vi "Conversion umToFs.vi"(8 "error in (no error)":errorcluster caption="entrée d'erreur (pas d'erreur)", 10 "um":dbl, 11 "UI SA en entrée":refnum<class "UI SmarAct.lvclass">) -> (0 "error out":errorcluster caption="sortie d'erreur", 2 "Fs":ext, 3 "UI SA en sortie":refnum<class "UI SmarAct.lvclass">)   [LabVIEW 2024, in "UI SmarAct.lvclass"]
uses:
  UI SmarAct.lvclass
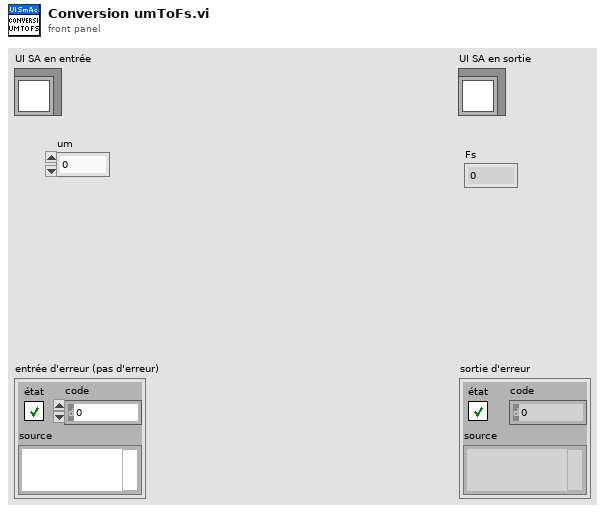
[diagram p1: front panel]
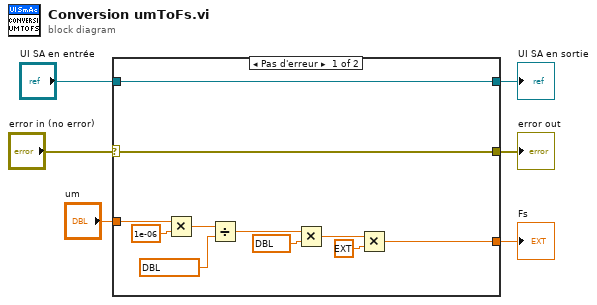
[diagram p0: block diagram]
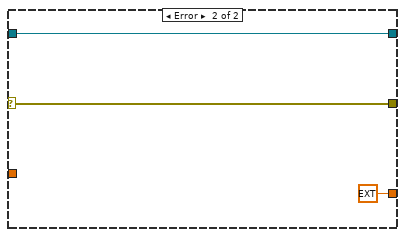
[diagram p2: hidden frame]
diagram:
  n1 = case shown="Pas d'erreur" "error in (no error)" {
    selector: "error in (no error)" -> [w16 w20]
    tunnel: [w16 w20] -> w5
    tunnel: [w17 w19] -> w3
    tunnel: "UI SA en entrée" -> [w17 w19]
    tunnel: "um" -> [w10 _]
    tunnel: [w8 ext 0.0] -> w1
    frame No Error {
      n2 = Multiply(x=w10, y=1e-06) -> (x*y=w11:dbl)
      n3 = Divide(x=w11, y=ext[unit] 300000000.0) -> (x/y=w15:ext[unit])
      n4 = Multiply(x=w15, y=ext[unit] 1000000000000000.0) -> (x*y=w9:ext)
      n5 = Multiply(x=w9, y=ext 2.0) -> (x*y=w8:ext)
    }
    frame Error {
    }
  }
  "error out" <- w5
  "UI SA en sortie" <- w3
  "Fs" <- w1
